vi "set_stringGenerator.vi"(8 "error in (no error)":errorcluster, 10 "subcomponents.stringGenerator":refnum<class "GenericStringGenerator.lvclass">, 11 "StimulatorAK101022TCP in":refnum<class "StimulatorAK101022TCP.lvclass">) -> (0 "error out":errorcluster, 3 "StimulatorAK101022TCP out":refnum<class "StimulatorAK101022TCP.lvclass">)   [LabVIEW 2010, in "StimulatorAK101022TCP.lvclass"]
uses:
  StimulatorAK101022TCP.lvclass
  StringGenerator/GenericStringGenerator/GenericStringGenerator/GenericStringGenerator.lvclass
  StimulatorAK101022TCP.lvclass/StimulatorAK101022TCP.ctl
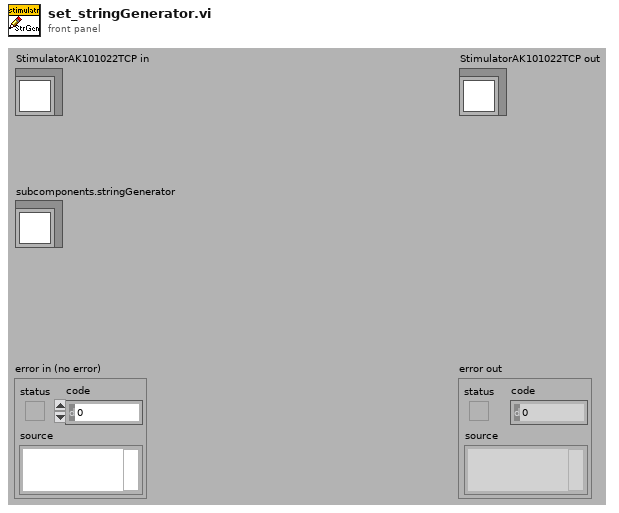
[diagram p1: front panel]
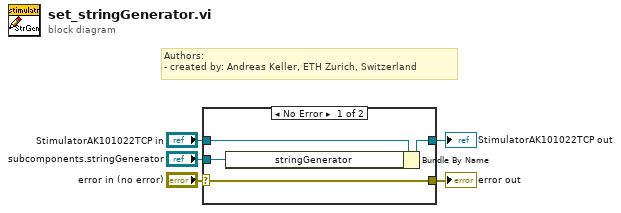
[diagram p0: block diagram]
diagram:
  # "Authors: \n- created by: Andreas Keller, ETH Zurich, Switzerland"
  n1 = case shown="No Error" "error in (no error)" {
    selector: "error in (no error)" -> [w9 w11]
    tunnel: [w9 w11] -> w4
    tunnel: [w7 w10] -> w2
    tunnel: "StimulatorAK101022TCP in" -> [w8 w10]
    tunnel: "subcomponents.stringGenerator" -> [w6 _]
    frame No Error {
      n2 = Bundle By Name(cluster=w8, "stringGenerator"=w6) -> (w7:refnum<class "StimulatorAK101022TCP.lvclass">)
    }
    frame Error {
    }
  }
  "error out" <- w4
  "StimulatorAK101022TCP out" <- w2
